vi "StringArrayToSet.vi"(11 "String Array":string[](array[string])) -> (3 "Set":set{string}(c389))   [LabVIEW 2021]
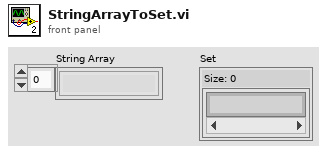
[diagram p1: front panel]
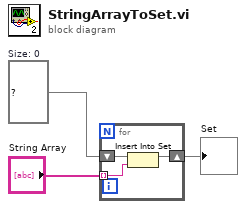
[diagram p0: block diagram]
diagram:
  w2 = set{string} {}  # Size: 0
  n1 = for {
    tunnel: "String Array" -> [w5] mode=indexing
    shift-right: [w4] -> w3
    shift-left: w2 -> [w6]
    n2 = Insert Into Set(10:w5, 11:w6) -> (3:w4:set{string})  [unwired: 1 out]
  }
  "Set" <- w3
